vi "Power Of X - CM,I.vi"(1 "Complex Matrix A":T1, 2 "Power n":i32) -> (0 "A^n":T1)   [LabVIEW 2017, in "NI_Matrix.lvlib"]
doc: "Computes the nth power of the input matrix."
uses:
  NI_Matrix.lvlib
  ComplexMatrix.ctl
  Complex Matrix Power.vi
  NI_AALBase.lvlib
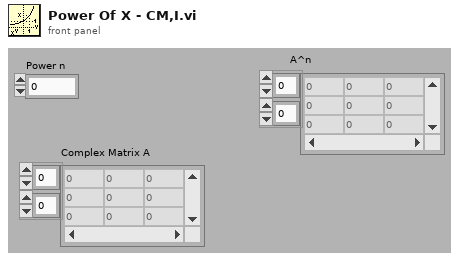
[diagram p1: front panel]
types:
  T1 = typedef "NI_Matrix.lvlib/ComplexMatrix.ctl" = cdb[][]
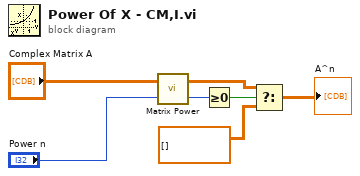
[diagram p0: block diagram]
diagram:
  n1 = call-poly "Matrix Power.vi"("n"="Power n", "Input Matrix"="Complex Matrix A") -> ("error"=w2:i32, "Matrix Power"=w1:T1)
  n2 = Greater Or Equal To 0?(x=w2) -> (x >= 0?=w7:bool)
  n3 = Select(t=w1, s=w7, f=T1 [] ("A^n")) -> (s? t:f=→"A^n":T1)
